vi "PF_Fitting.vi"(7 "Interpolation Range":dbl=0.37, 8 "Extrema Array":T1(array[cluster]), 10 "Intensity Array":dbl[](array[numeric])) -> (0 "Intensity":cluster{dbl[], dbl[]}[](graph), 1 "yFit":dbl[](array[numeric]), 2 "xFit":dbl[](array[numeric]))   [LabVIEW 2020]
uses:
  <vilib>/Analysis/1siggen.llb/Ramp Pattern by Samples.vi
  <vilib>/Analysis/NI_AALBase.lvlib
  <vilib>/Analysis/NI_AALPro.lvlib
panel:
  in  "extremum":T2={"type"=enum."maximum", "x"=0, "y"=0.0} {"y" format="%.2f"}
  # "Phase Fitter: Fitting"
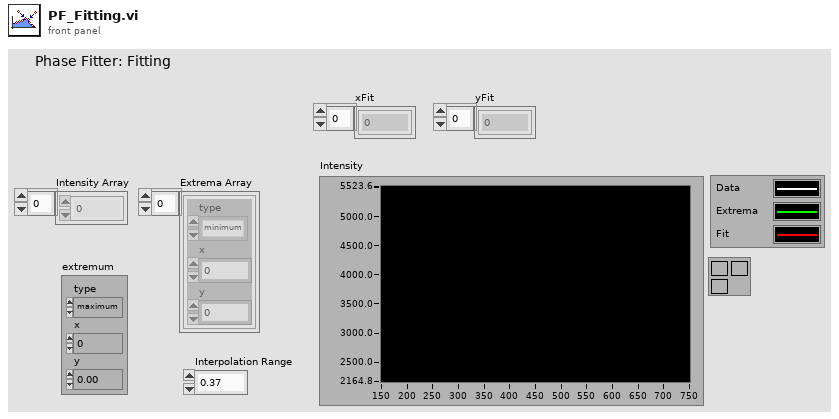
[diagram p1: front panel]
types:
  T1 = cluster{"type":enum16{"minimum", "maximum"}, "x":i32, "y":dbl}[]
  T2 = cluster{"type":enum16{"minimum", "maximum"}, "x":i32, "y":dbl}
  T3 = cluster{"Ramp Pattern":dbl[], "Intensity Array":dbl[]}
  T4 = cluster{"Ramp Pattern":dbl[], "Best Polynomial Fit":dbl[]}[]
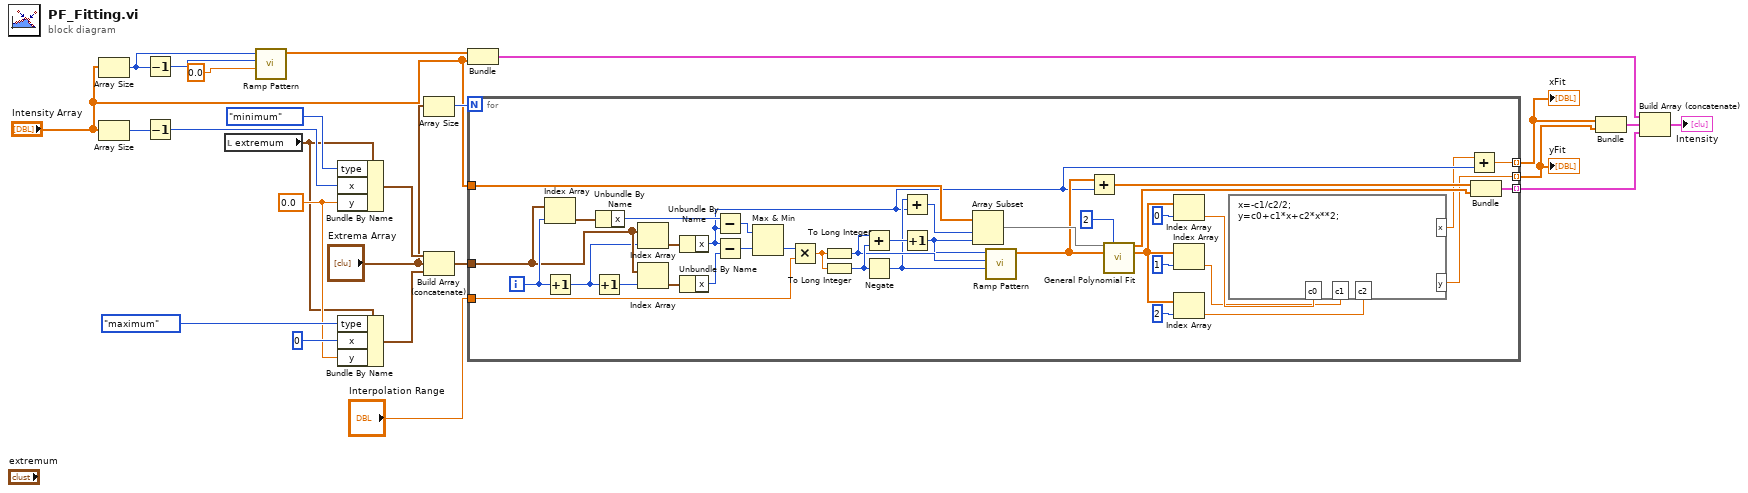
[diagram p0: block diagram]
diagram:
  w18 = 0.0
  n1 = Array Size(array="Intensity Array") -> (size(s)=w6:i32)
  n2 = Array Size(array="Intensity Array") -> (size(s)=w12:i32)
  n3 = Decrement(x=w6) -> (x-1=w5:i32)
  n4 = Decrement(x=w12) -> (x-1=w20:i32)
  n5 = local read "extremum"() -> (w16:T2)
  n6 = call-poly <vilib>:"Ramp Pattern.vi"("start"=0.0, "end"=w5, "samples"=w6) -> ("Ramp Pattern"=w3:dbl[])  [unwired: 7 in, 1 out]
  n7 = Bundle By Name(cluster=w16, "type"=enum16{"minimum", "maximum"}."minimum" ("Bundle Element"), "x"=w20, "y"=w18) -> (w17:T2)
  n8 = Bundle By Name(cluster=w16, "type"=enum16{"minimum", "maximum"}."maximum" ("Bundle Element"), "x"=0 ("Input Element"), "y"=w18) -> (w15:T2)
  n9 = Array Size(array="Extrema Array") -> (size(s)=w14:i32)
  n10 = Build Array (concatenate)(w17, "Extrema Array", w15) -> (w13:T1)
  n11 = Bundle("Ramp Pattern"=w3, "Intensity Array"="Intensity Array") -> (w1:T3)  [unwired: 1 out]
  n12 = for {
    N: w14 -> [_]
    tunnel: "Intensity Array" -> [w62]
    tunnel: [w58] -> w9 mode=indexing
    tunnel: w13 -> [w55]
    tunnel: "Interpolation Range" -> [w32]
    tunnel: [w25] -> w10 mode=indexing
    tunnel: [w28] -> w11 mode=indexing
    i -> [w56]
    n13 = Index Array(array=w55, index=w56) -> (element=w42:T2)
    n14 = Increment(x=w56) -> (x+1=w54:i32)
    n15 = Increment(x=w54) -> (x+1=w53:i32)
    n16 = Unbundle By Name(w42) -> ("x"=w40:i32)
    n17 = Index Array(array=w55, index=w54) -> (element=w33:T2)
    n18 = Index Array(array=w55, index=w53) -> (element=w41:T2)
    n19 = Unbundle By Name(w33) -> ("x"=w29:i32)
    n20 = Unbundle By Name(w41) -> ("x"=w39:i32)
    n21 = Subtract(x=w40, y=w29) -> (x-y=w31:i32)
    n22 = Subtract(x=w29, y=w39) -> (x-y=w52:i32)
    n23 = Max & Min(x=w31, y=w52) -> (min(x,y)=w49:i32)  [unwired: 1 out]
    n24 = Multiply(x=w49, y=w32) -> (x*y=w30:dbl)
    n25 = To Long Integer(number=w30) -> (32bit integer=w38:i32)
    n26 = To Long Integer(number=w30) -> (32bit integer=w51:i32)
    n27 = Add(x=w38, y=w51) -> (x+y=w50:i32)
    n28 = Negate(x=w51) -> (-x=w37:i32)
    n29 = Add(x=w37, y=w29) -> (x+y=w36:i32)
    n30 = Increment(x=w50) -> (x+1=w35:i32)
    n31 = Array Subset(array=w62, index=w36, length=w35) -> (w61:dbl[])
    n32 = call-poly <vilib>:"Ramp Pattern.vi"("start"=w37, "end"=w38, "samples"=w35) -> ("Ramp Pattern"=w57:dbl[])  [unwired: 7 in, 1 out]
    n33 = Add(x=w57, y=w29) -> (x+y=w60:dbl[])
    n34 = call <vilib>:"General Polynomial Fit.vi"("Y"=w61, "polynomial order"=2, "X"=w57) -> ("Best Polynomial Fit"=w59:dbl[], "Polynomial Coefficients"=w34:dbl[])  [unwired: 9 in, 2 out]
    n35 = Index Array(array=w34, index=0 ("Index")) -> (element=w45:dbl)
    n36 = Index Array(array=w34, index=1 ("Index")) -> (element=w44:dbl)
    n37 = Index Array(array=w34, index=2 ("Index")) -> (element=w43:dbl)
    n38 = formula code="x=-c1/c2/2;\ny=c0+c1*x+c2*x**2;"("c0"=w45, "c2"=w43, "c1"=w44) -> ("x"=w26:dbl, "y"=w25:dbl)
    n39 = Add(x=w26, y=w29) -> (x+y=w28:dbl)
    n40 = Bundle(w60, "Best Polynomial Fit"=w59) -> (w58:cluster{dbl[], "Best Polynomial Fit":dbl[]})  [unwired: 1 out]
  }
  "yFit" <- w10
  "xFit" <- w11
  n41 = Bundle(w11, w10) -> (w23:cluster{dbl[], dbl[]})  [unwired: 1 out]
  n42 = Build Array (concatenate)(w1, w23, w9) -> (→"Intensity":T4)
